vi "Create Injectors.vi"(7 "Max Shots":T1(ring)=enum."1", 8 "error in (no error)":errorcluster, 9 "Stages":string[](array[string])=["Boost", "Battery", "Off"], 10 "NewVal":path, 11 "Item Ref in":T2 format="%.0x") -> (0 "error out":errorcluster, 3 "Section Ref out":T2 format="%.0x")   [LabVIEW 2015, in "Fuel Injection Addon System Explorer.lvlib"]
uses:
  Fuel Injection Addon System Explorer.lvlib
  <vilib>/NI Veristand/Custom Device API/Custom Device Item Ref.ctl
  Shared/Constants.vi
  <vilib>/NI Veristand/Custom Device API/Set Item Property (Path).vi
  <vilib>/NI VeriStand/Custom Device API/Custom Device API.lvlib
  Shared/Fuel Injection Addon Shared.lvlib
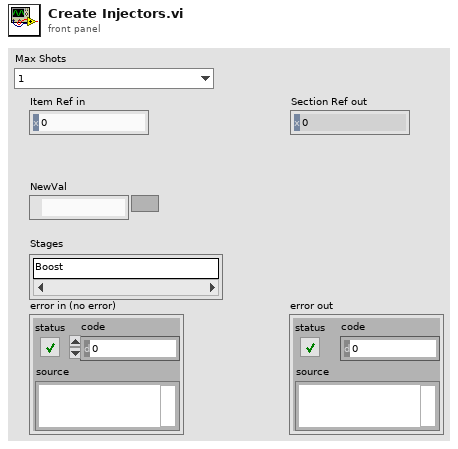
[diagram p1: front panel]
types:
  T1 = enum16{"0", "1", "2", "3", "4", "5", "6", "7", "8"}
  T2 = typedef "Custom Device API.lvlib/Custom Device Item Ref.ctl" = u64
  T3 = typedef "Fifo_DMA_Config.ctl" = cluster{"Name":string, "Depth":u32, "Write? (Deprecated:Use Implementation)":bool, "Physical Channel":u32, "Base Address":u32, "Data Width":u32, "Data Type":T4, "FXP Properties":variant, "Write Window Address":u32, "Implementation":T5, "Control Set":u32}
  T4 = typedef "niFpgaDataTypeControl.ctl" = enum32{"Boolean", "I8", "I16", "I32", "I64", "U8", "U16", "U32", "U64", "FXP", "CustomControl", "SGL"}
  T5 = typedef "niFpgaDmaChannelImplementation.ctl" = enum16{"niFpgaTargetToHost", "niFpgaHostToTarget", "niFpgaPeerToPeerWriter", "niFpgaPeerToPeerReader", "niCoreTargetToHost", "niCoreHostToTarget"}
  T6 = typedef "niFpgaBitfileStructure_VI.ctl" = cluster{"Name":string, "RegisterMap":T7[], "Icon":T12}
  T7 = typedef "nirviControlStructure.ctl" = cluster{"Name":string, "Hidden":bool, "Indicator":bool, "Flattened Type":string, "Grouping":cluster{"Grouped":bool, "Member Names":string[], "Member IDs":u32[]}, "Address":u32, "Size":u32, "Class":u32, "Internal":bool, "Typedef":T8, "ID":u32, "Bidirectional":bool, "Synchronous":bool, "Mechanical Action":T9, "Sub Controls":T10[], "Access May Timeout":bool, "Register Node":bool}
  T8 = typedef "nirviTypdefDescription.ctl" = cluster{"Typedef":bool, "Path":path}
  T9 = typedef "nirviMechanicalAction.ctl" = enum8{"Switch When Pressed", "Switch When Released", "Switch Until Released", "Latch When Pressed", "Latch When Released", "Latch Until Released"}
  T10 = typedef "nirviSubControlStructure.ctl" = cluster{"Name":string, "flattened Type":string, "Cluster Information":T11, "Typedef":T8}
  T11 = typedef "nirviClusterElementControl.ctl" = cluster{"Name Hierarchy":string[], "Item Order":u32[]}
  T12 = typedef "imagedata.ctl" = cluster{"image type":i32, "image depth":i32, "image":u8[], "mask":u8[], "colors":u32[], "Rectangle":cluster{"left":i16, "top":i16, "right":i16, "bottom":i16}}
  T13 = typedef "Fuel Injection Addon Shared.lvlib/Register.Info.ctl" = cluster{"Name":string, "Data Type":T14, "Default Value":variant}
  T14 = typedef "Fuel Injection Addon Shared.lvlib/FPGA Data Types.ctl" = enum8{"<Null>", "Injector.Core.Setting", "Injector.Global.Setting", "Injector.Mux.Setting", "Injector.Timing"}
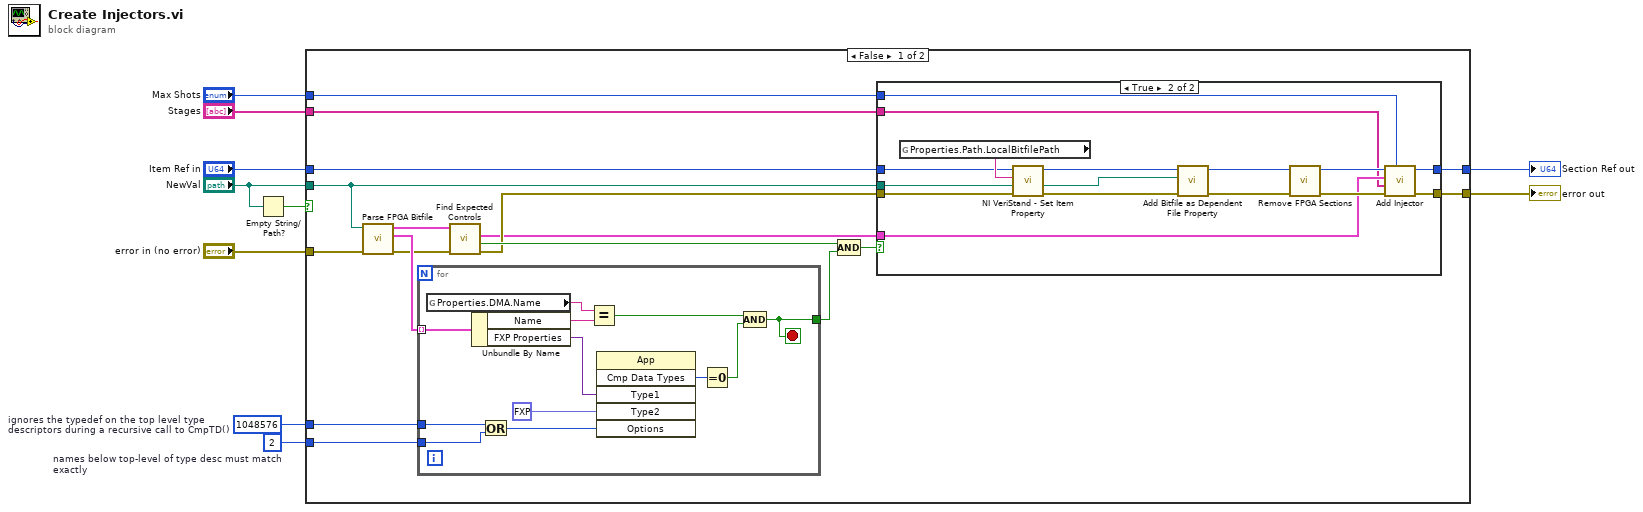
[diagram p0: block diagram]
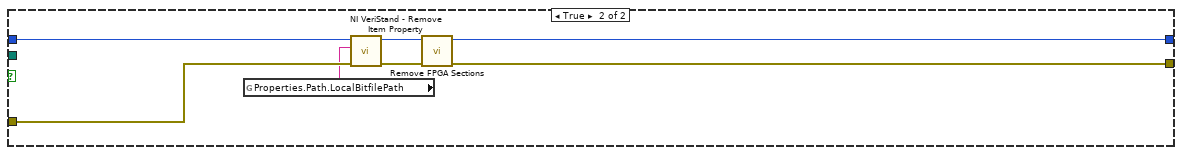
[diagram p3: hidden frame]
diagram:
  w3 = 2  # names below top-level of type desc must match exactly
  w4 = 1048576  # ignores the typedef on the top level type descriptors during a recursive call to CmpTD()
  n1 = Empty String/Path?(string/path="NewVal") -> (empty?=w8:bool)
  n2 = case shown="False" w8 {
    tunnel: "NewVal" -> [w18 _]
    tunnel: "error in (no error)" -> [w23 w62]
    tunnel: [w15 w58] -> w10
    tunnel: [w16 w57] -> w9
    tunnel: "Item Ref in" -> [w19 w63]
    tunnel: w4 -> [w25 _]
    tunnel: w3 -> [w24 _]
    tunnel: "Stages" -> [w12 _]
    tunnel: "Max Shots" -> [w11 _]
    frame False {
      n3 = call "Parse FPGA Bitfile.vi"("error in (no error)"=w23, "Path"=w18) -> ("error out"=w20:errorcluster, "DMA configuration array"=w22:T3[], "vi info"=w21:T6)  [unwired: 7 in]
      n4 = for {
        tunnel: w22 -> [w56] mode=indexing
        tunnel: [w52] -> w27
        tunnel: w25 -> [w47]
        tunnel: w24 -> [w46]
        stop <- w52 stop-if-true
        n5 = global read "Constants.vi" "Properties.DMA.Name"() -> (w54:string)
        n6 = Unbundle By Name(w56) -> ("Name"=w55:string, "FXP Properties"=w45:variant)
        n7 = Or(x=w47, y=w46) -> (x .or. y?=w51:i32)
        n8 = Equal?(x=w54, y=w55) -> (x = y?=w53:bool)
        n9 = invoke class="App" method="Cmp Data Types"("Type1"=w45, "Type2"=fxp<+/-,32,8> 0.0, "Options"=w51) -> ("Compare Data Types"=w49:i32)  [unwired: 3 in, 5 out]
        n10 = Equal To 0?(x=w49) -> (x = 0?=w48:bool)
        n11 = Compound Arithmetic op=AND(w53, w48) -> (w52:bool)
      }
      n12 = call "Find Expected Controls.vi"("error in"=w20, "vi info"=w21) -> ("error out"=w17:errorcluster, "Use?"=w26:bool, "Controls"=w13:T13[])  [unwired: 6 in, 1 out]
      n13 = Compound Arithmetic op=AND(w26, w27) -> (w14:bool)
      n14 = case shown="True" w14 {
        tunnel: w19 -> [w28 w38]
        tunnel: w18 -> [_ w41]
        tunnel: w17 -> [w29 w40]
        tunnel: [w28 w32] -> w16
        tunnel: [w29 w35] -> w15
        tunnel: w13 -> [_ w34]
        tunnel: w12 -> [_ w31]
        tunnel: w11 -> [_ w30]
        frame False {
        }
        frame True {
          n15 = global read "Constants.vi" "Properties.Path.LocalBitfilePath"() -> (w42:string)
          n16 = call-poly <vilib>:"NI VeriStand - Set Item Property.vi"("error in (no error)"=w40, "Value"=w41, "Property Name"=w42, "Item Ref in"=w38) -> ("error out"=w39:errorcluster, "Item Ref out"=w37:T2)  [unwired: 5 in, 1 out]
          n17 = call "Add Bitfile as Dependent File Property.vi"("error in"=w39, "Local bitfile path"=w41, "Device Item Ref"=w37) -> ("error out"=w43:errorcluster, "Device Item Ref out"=w44:T2)  [unwired: 7 in]
          n18 = call "Remove FPGA Sections.vi"("error in (no error)"=w43, "Item Ref in"=w44) -> ("error out"=w36:errorcluster, "Item Ref out"=w33:T2)  [unwired: 8 in]
          n19 = call "Add Injector.vi"("Max Shots"=w30, "error in (no error)"=w36, "Stages"=w31, "Controls"=w34, "Item Ref"=w33) -> ("error out"=w35:errorcluster, "Item Ref out"=w32:T2)  [unwired: 5 in]
        }
      }
    }
    frame True {
      n20 = global read "Constants.vi" "Properties.Path.LocalBitfilePath"() -> (w61:string)
      n21 = call <vilib>:"NI VeriStand - Remove Item Property.vi"("error in (no error)"=w62, "Property Name"=w61, "Item Ref in"=w63) -> ("error out"=w59:errorcluster, "Item Ref out"=w60:T2)  [unwired: 6 in, 1 out]
      n22 = call "Remove FPGA Sections.vi"("error in (no error)"=w59, "Item Ref in"=w60) -> ("error out"=w58:errorcluster, "Item Ref out"=w57:T2)  [unwired: 8 in]
    }
  }
  "error out" <- w10
  "Section Ref out" <- w9
